vi "GetHomingStatus.vi"(7 "ArmID":i32) -> (0 "Homing XYZ Stage Done":bool, 1 "Homing Tool Done":bool, 2 "Homing Arm Done":bool)   [LabVIEW 2016]
uses:
  EyeRobotDLL.dll
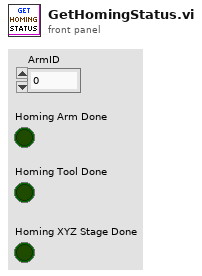
[diagram p1: front panel]
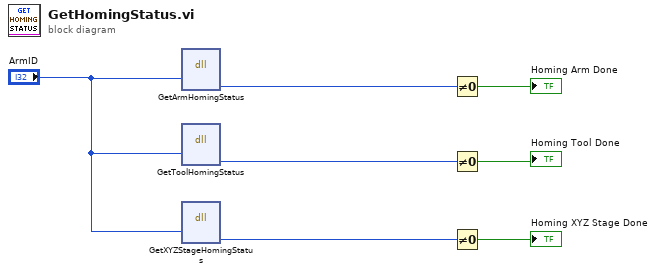
[diagram p0: block diagram]
diagram:
  n1 = dll-call lib="D:/Kevin/IRISS V2 dev/Host Demo/Functions/EyeRobotDLL.dll" fn="GetArmHomingStatus"("id"="ArmID") -> ("status"=w5:u8)  [unwired: 6 in, 2 out]
  n2 = dll-call lib="D:/Kevin/IRISS V2 dev/Host Demo/Functions/EyeRobotDLL.dll" fn="GetToolHomingStatus"("id"="ArmID") -> ("status"=w4:u8)  [unwired: 6 in, 2 out]
  n3 = dll-call lib="D:/Kevin/IRISS V2 dev/Host Demo/Functions/EyeRobotDLL.dll" fn="GetXYZStageHomingStatus"("id"="ArmID") -> ("status"=w3:u8)  [unwired: 6 in, 2 out]
  n4 = Not Equal To 0?(x=w5) -> (x != 0?=→"Homing Arm Done":bool)
  n5 = Not Equal To 0?(x=w4) -> (x != 0?=→"Homing Tool Done":bool)
  n6 = Not Equal To 0?(x=w3) -> (x != 0?=→"Homing XYZ Stage Done":bool)
